vi "Read Volume Dispensed.vi"(7 "Pump ID (0:A)":T1, 8 "error in (no error)":errorcluster, 11 "VISA resource in":refnum<visa-resource-name>) -> (0 "error out":errorcluster, 2 "microliters":dbl, 3 "VISA resource out":refnum<visa-resource-name>)   [LabVIEW 2020, in "Global FIA milliGAT.lvlib"]
doc: "Read the position of the pump relative to to when the pump move started."
uses:
  <instrlib>/RxnRover/Global FIA milliGAT 3.14/Global FIA milliGAT.lvlib
  <instrlib>/RxnRover/Global FIA milliGAT 3.14/Public/Utility/Pump Address.ctl
  <instrlib>/RxnRover/Global FIA milliGAT 3.14/Private/Pump Parameter.ctl
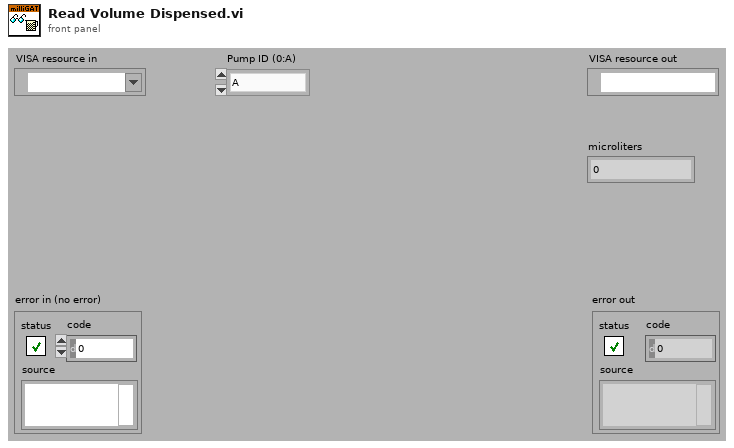
[diagram p1: front panel]
types:
  T1 = typedef "Global FIA milliGAT.lvlib/Pump Address.ctl" = enum16{"A", "B", "C", "D", "E", "F", "G", "H", "I", "J", "K", "L", "M", "N", "O", "P", "Q", "R", "S", "T", "U", "V", "W", "X", "Y", "Z", "a", "b", "c", "d", "e", "f", "g", "h", "i", "j", "k", "l", "m", "n", "o", "p", "q", "r", "s", "t", "u", "v", "w", "x", "y", "z", "0", "1", "2", "3", "4", "5", "6", "7", "8", "9"}
  T2 = typedef "Global FIA milliGAT.lvlib/Pump Parameter.ctl" = enum16{"Enabled", "EU", "EU Calibration Factor", "Fixed Asp or Disp", "Starting Position", "Starting Flow", "Peak Flow", "Flow Acceleration", "Flow Deceleration", "Session Volume", "Max Pressure", "Backlash (usteps)", "BL Calibration Factor", "BL Correction Enabled", "Min Flow", "Max Flow", "Min Acceleration", "Max Acceleration", "Service Volume", "Life Volume"}
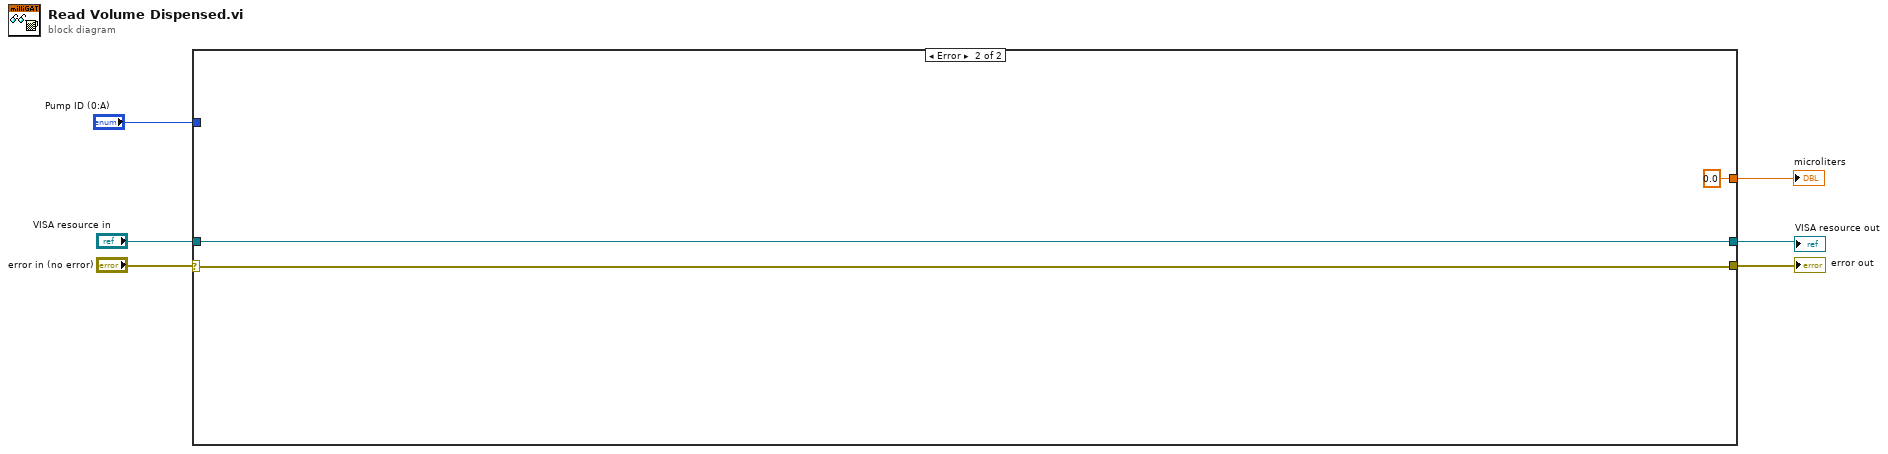
[diagram p0: block diagram]
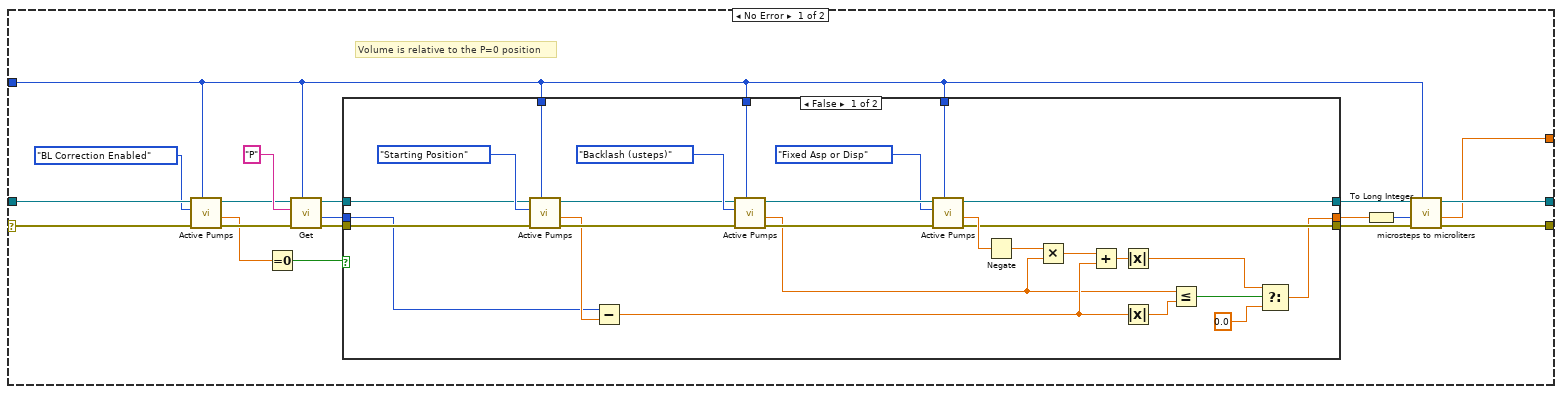
[diagram p2: hidden frame]
diagram:
  n1 = case shown="Error" "error in (no error)" {
    selector: "error in (no error)" -> [w7 w58]
    tunnel: [w24 w57] -> w6
    tunnel: [w23 w58] -> w5
    tunnel: "VISA resource in" -> [w22 w57]
    tunnel: "Pump ID (0:A)" -> [w11 _]
    tunnel: [w9 0.0 ("Microliters")] -> w2
    frame No Error {
      # "Volume is relative to the P=0 position"
      n2 = call <instrlib>:"Active Pumps.vi"("Pump ID (0:A)"=w11, "error in (no error)"=w7, "Parameter"=Pump_Parameter."BL Correction Enabled", "VISA resource in"=w22) -> ("error out"=w19:errorcluster, "Value out"=w18:dbl, "VISA resource out"=w21:refnum<visa-resource-name>)  [unwired: 4 in, 1 out]
      n3 = Equal To 0?(x=w18) -> (x = 0?=w17:bool)
      n4 = call <instrlib>:"Get.vi"("Pump ID (0:A)"=w11, "error in (no error)"=w19, "Parameter"="P" ("Parameter or Flag Name"), "VISA resource in"=w21) -> ("error out"=w16:errorcluster, "Value"=w12:i32, "VISA resource out"=w14:refnum<visa-resource-name>)  [unwired: 5 in]
      n5 = case shown="False" w17 {
        tunnel: w16 -> [w50 w55]
        tunnel: [w28 w55] -> w15
        tunnel: w14 -> [w49 w54]
        tunnel: [w29 w54] -> w13
        tunnel: w12 -> [w45 w53]
        tunnel: [w27 w53] -> w10
        tunnel: w11 -> [w47 _]
        tunnel: w11 -> [w43 _]
        tunnel: w11 -> [w40 _]
        frame False {
          n6 = call <instrlib>:"Active Pumps.vi"("Pump ID (0:A)"=w47, "error in (no error)"=w50, "Parameter"=Pump_Parameter."Starting Position", "VISA resource in"=w49) -> ("error out"=w48:errorcluster, "Value out"=w46:dbl, "VISA resource out"=w44:refnum<visa-resource-name>)  [unwired: 4 in, 1 out]
          n7 = Subtract(x=w45, y=w46) -> (x-y=w35:dbl)
          n8 = call <instrlib>:"Active Pumps.vi"("Pump ID (0:A)"=w43, "error in (no error)"=w48, "Parameter"=Pump_Parameter."Backlash (usteps)", "VISA resource in"=w44) -> ("error out"=w41:errorcluster, "Value out"=w33:dbl, "VISA resource out"=w42:refnum<visa-resource-name>)  [unwired: 4 in, 1 out]
          n9 = call <instrlib>:"Active Pumps.vi"("Pump ID (0:A)"=w40, "error in (no error)"=w41, "Parameter"=Pump_Parameter."Fixed Asp or Disp", "VISA resource in"=w42) -> ("error out"=w28:errorcluster, "Value out"=w38:dbl, "VISA resource out"=w29:refnum<visa-resource-name>)  [unwired: 4 in, 1 out]
          n10 = Negate(x=w38) -> (-x=w37:dbl)
          n11 = Multiply(x=w37, y=w33) -> (x*y=w36:dbl)
          n12 = Add(x=w36, y=w35) -> (x+y=w34:dbl)
          n13 = Absolute Value(x=w34) -> (abs(x)=w31:dbl)
          n14 = Absolute Value(x=w35) -> (abs(x)=w30:dbl)
          n15 = Less Or Equal?(x=w33, y=w30) -> (x <= y?=w32:bool)
          n16 = Select(t=w31, s=w32, f=0.0) -> (s? t:f=w27:dbl)
        }
        frame True {
        }
      }
      n17 = To Long Integer(number=w10) -> (32bit integer=w8:i32)
      n18 = call <instrlib>:"microsteps to microliters.vi"("Pump ID (0:A)"=w11, "error in (no error)"=w15, "Microsteps (0)"=w8, "VISA resource in"=w13) -> ("error out"=w23:errorcluster, "Microliters"=w9:dbl, "VISA resource out"=w24:refnum<visa-resource-name>)  [unwired: 5 in]
    }
    frame Error {
    }
  }
  "VISA resource out" <- w6
  "error out" <- w5
  "microliters" <- w2
